vi "lasernoise.vi"() -> ()   [LabVIEW 2013]
uses:
  <vilib>/express/express analysis/Spectral/Block/exnSpectralBlock spectral measurements RMS poly.vi
  <vilib>/express/express analysis/Spectral/Block/exnSpectralBlock spectral measurements RMS DDT.vi
  <vilib>/express/express analysis/Spectral/XNode/ExpressSpectralMeasurementsBlockNode.xnode
  <vilib>/Analysis/NI_AALBase.lvlib
panel:
  in  "number of samples":i32=10000
  out "STDev":dbl
  out "MEAN":dbl
  in  "Meas":bool
  in  "Quit":bool
  out "FFT":dynamicdata(graph)
  out "data":dynamicdata(graph) caption="TIME"
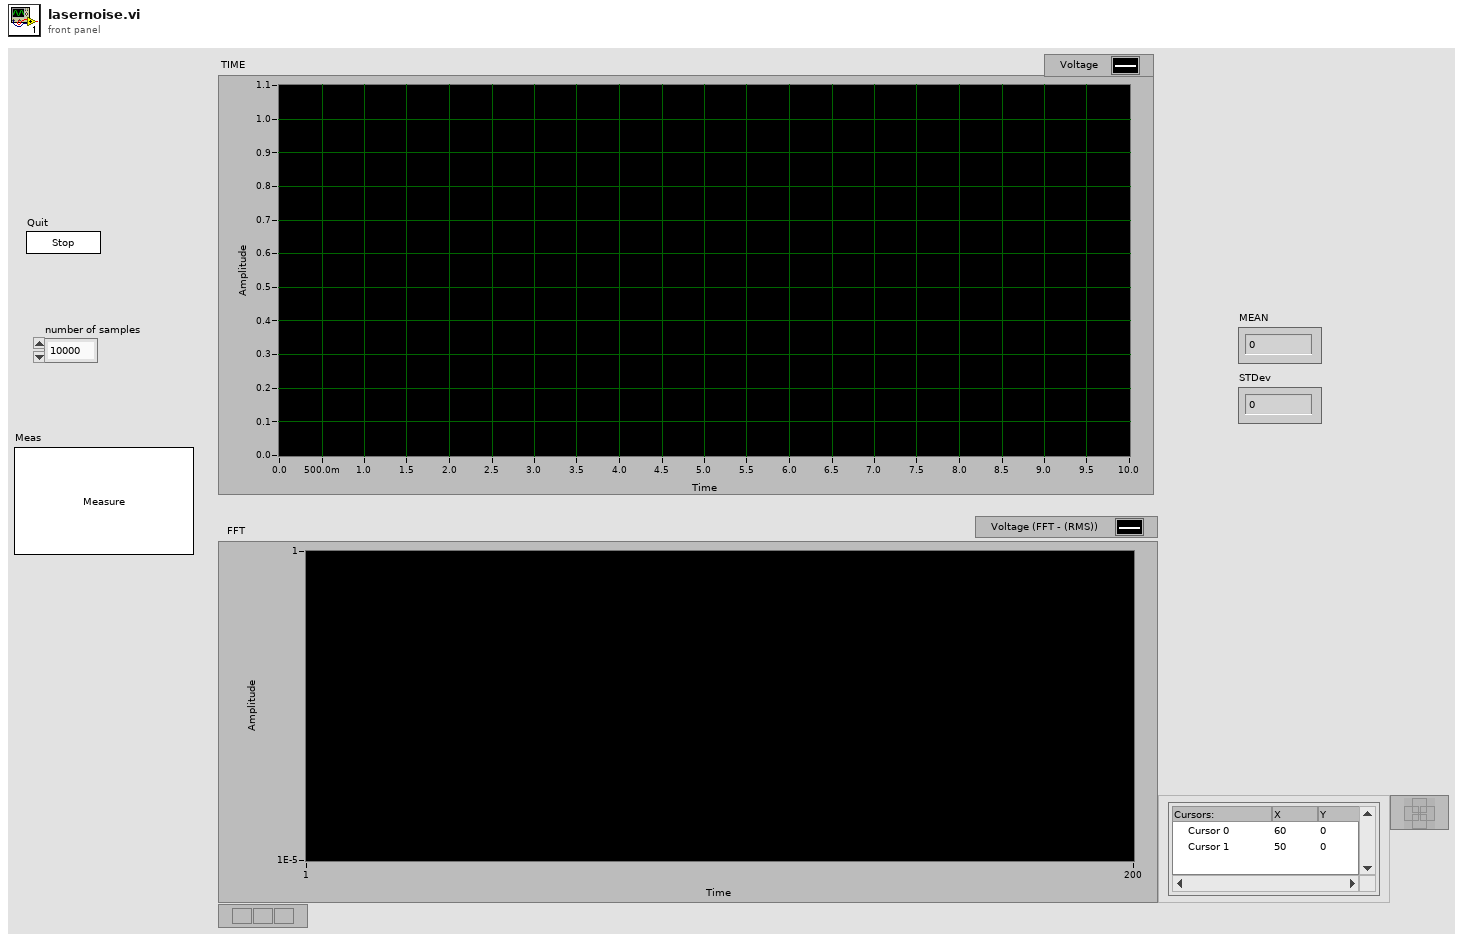
[diagram p1: front panel]
types:
  T1 = cluster{"averaging mode":u16, "weighting mode":u16, "number of averages":u32}
  T2 = cluster{"dB On (F)":bool, "unwrap phase (F)":bool, "convert to degree (F)":bool}
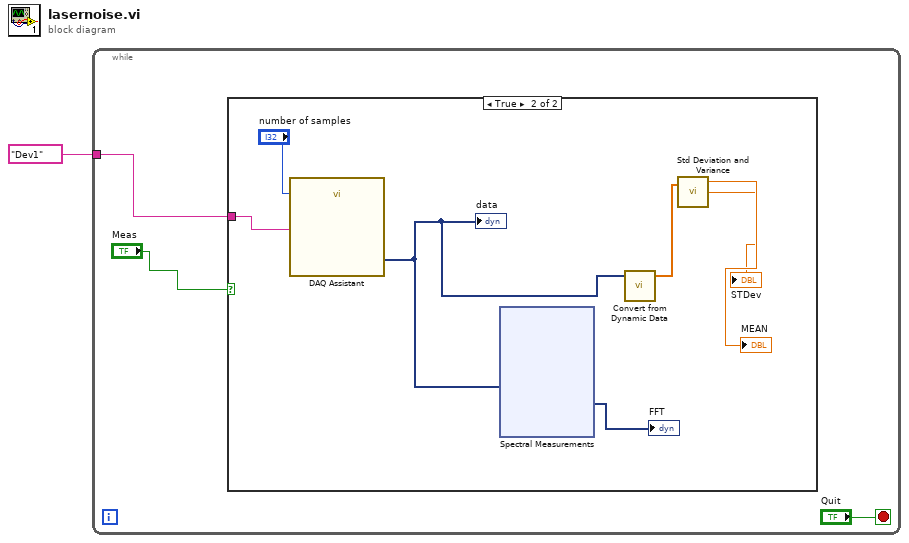
[diagram p0: block diagram]
diagram:
  n1 = while {
    tunnel: tag "Dev1" ("device name") -> [w4]
    stop <- "Quit" stop-if-true
    n2 = case shown="True" "Meas" {
      tunnel: w4 -> [_ w11]
      frame False {
      }
      frame True {
        n3 = call "DAQ Assistant"("number of samples"="number of samples", "device name"=w11) -> ("data"=w9:dynamicdata)  [unwired: 15 in, 2 out]
        "data" <- w9
        n4 = xnode "Spectral Measurements"("Signals"=w9) -> ("FFT - (RMS)"=→"FFT":dynamicdata)  [unwired: 1 in, 2 out]
        n5 = call "Convert from Dynamic Data"("Dynamic Data Type"=w9) -> ("Array"=w6:dbl[])  [unwired: 3 in]
        n6 = call <vilib>:"Std Deviation and Variance.vi"("X"=w6) -> ("mean"=→"MEAN":dbl, "standard deviation"=→"STDev":dbl)  [unwired: 1 in, 1 out]
      }
    }
  }
